vi "Tell No Relation.vi"(4 "Priority":bool, 7 "Actor in":refnum<class "Actor.lvclass">, 8 "Error in":errorcluster, 9 "Transport":refnum<class "Transport.lvclass">, 10 "Msg":refnum<class "Msg.lvclass">) -> (0 "Error out":errorcluster, 5 "Actor out":refnum<class "Actor.lvclass">)   [LabVIEW 2020, in "jettl.lvlib"]
uses:
  jettl.lvlib
  Msg/Msg.lvclass
  Actor/Actor.lvclass
  Transport/Transport.lvclass
  Teller Metadata/Teller Metadata.lvclass
  Relation.ctl
  Teller.ctl
  Read Self Attributes/Read Self Attributes.lvlib
  Read Self Attributes/UID.vi
  Read Self Attributes/Alias.vi
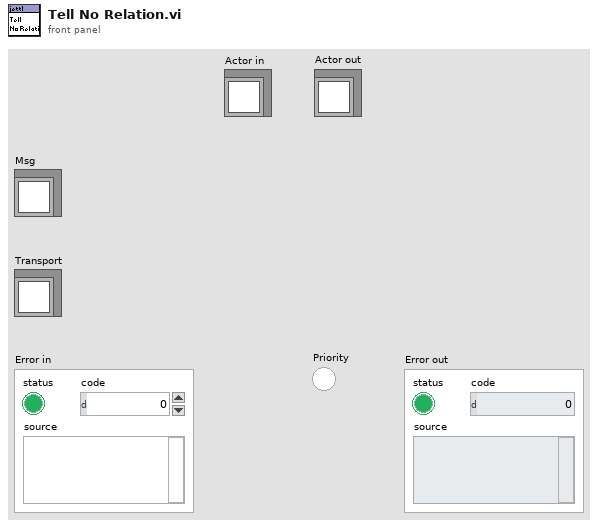
[diagram p1: front panel]
types:
  T1 = typedef "jettl.lvlib/Relation.ctl" = enum16{"Self", "Parent", "Child"}
  T2 = typedef "jettl.lvlib/Teller.ctl" = cluster{"Priority":bool, "Absolute Time":timestamp, "Relative Time":dbl, "UID":i32, "Alias":string, "Valid Relation":bool, "Relation":T1, "Called From Msg Library":bool, "Teller Metadata":refnum<class "Teller Metadata.lvclass">}
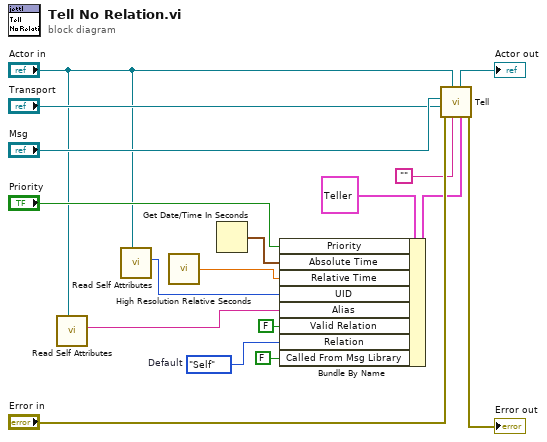
[diagram p0: block diagram]
diagram:
  w9 = Relation."Self"  # Default
  n1 = call-poly "Read Self Attributes.vi"("Actor in"="Actor in") -> ("Alias"=w6:string)  [unwired: 10 in]
  n2 = call-poly "Read Self Attributes.vi"("Actor in"="Actor in") -> ("UID"=w17:i32)  [unwired: 10 in]
  n3 = call <vilib>:"High Resolution Relative Seconds.vi"() -> ("relative seconds"=w1:dbl)
  n4 = Get Date/Time In Seconds() -> (seconds since 1Jan1904=w2:timestamp)
  n5 = Bundle By Name(cluster=T2 {"Priority"=FALSE, "Absolute Time"=timestamp(0 s since 1904-01-01), "Relative Time"=0.0, "UID"=0, "Alias"="", "Valid Relation"=FALSE, "Relation"=enum."Self", "Called From Msg Library"=FALSE, "Teller Metadata"=refnum} ("Teller Elements"), "Priority"="Priority", "Absolute Time"=w2, "Relative Time"=w1, "UID"=w17, "Alias"=w6, "Valid Relation"=FALSE, "Relation"=w9, "Called From Msg Library"=FALSE) -> (w4:T2)
  n6 = call "Tell.vi"("Teller"=w4, "Alias"="", "Actor in"="Actor in", "Error in"="Error in", "Transport"="Transport", "Msg"="Msg") -> ("Error out"=→"Error out":errorcluster, "Actor out"=→"Actor out":refnum<class "Actor.lvclass">)  [unwired: 4 in]
